vi "Enable All Axes.vi"(8 "error in (no error)":errorcluster, 11 "A3200 in":refnum<class "A3200.lvclass">) -> (0 "error out":errorcluster, 3 "A3200 out":refnum<class "A3200.lvclass">)   [LabVIEW 2016, in "A3200.lvclass"]
uses:
  A3200.lvclass
  A3200.lvclass/A3200.ctl
  Drivers/Aerotech A3200/Aerotech VIs.lvlib
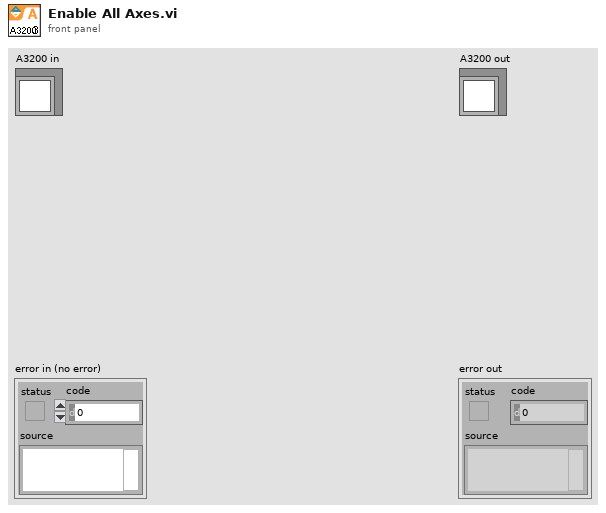
[diagram p1: front panel]
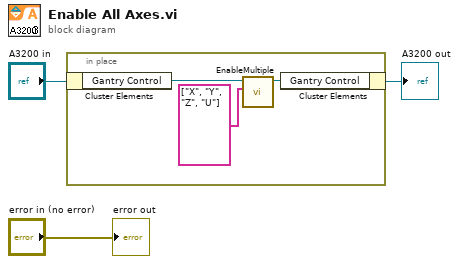
[diagram p0: block diagram]
diagram:
  n1 = in-place {
    n2 = in-place-cluster #1("A3200 in") -> ("Gantry Control"=w5:refnum<k24>)
    n3 = call "EnableMultiple.vi"("axis names"=string[] ["X", "Y", "Z", "U"], "controller in"=w5) -> ("controller out"=w4:refnum<k24>)  [unwired: 8 in, 1 out]
    n4 = in-place-cluster #1("Gantry Control"=w4) -> (→"A3200 out":refnum<class "A3200.lvclass">)
  }
  "error out" <- "error in (no error)"
